vi "Advance past replacable whitespace.vi"(7 "JSON":string, 9 "Offset":i32) -> (1 "Offset of first non-whitespace":i32)   [LabVIEW 2019, in "JSONtext.lvlib"]
doc: "Advance past only whitespace that can be used in a replacement\n-- no comments, as partial replacement will cause corupt JSON"
uses:
  JSONtext.lvlib
  Parsing State.ctl
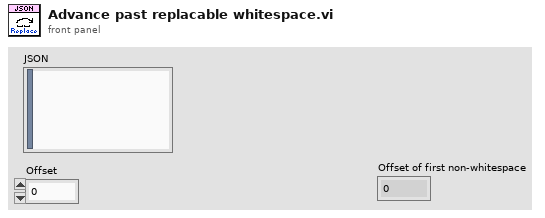
[diagram p1: front panel]
types:
  T1 = typedef "JSONtext.lvlib/Parsing State.ctl" = enum16{"Parser Error", "Object", "Array", "String", "Number/Other", "Leading Whitespace", "Object end", "Array end", "Value end"}
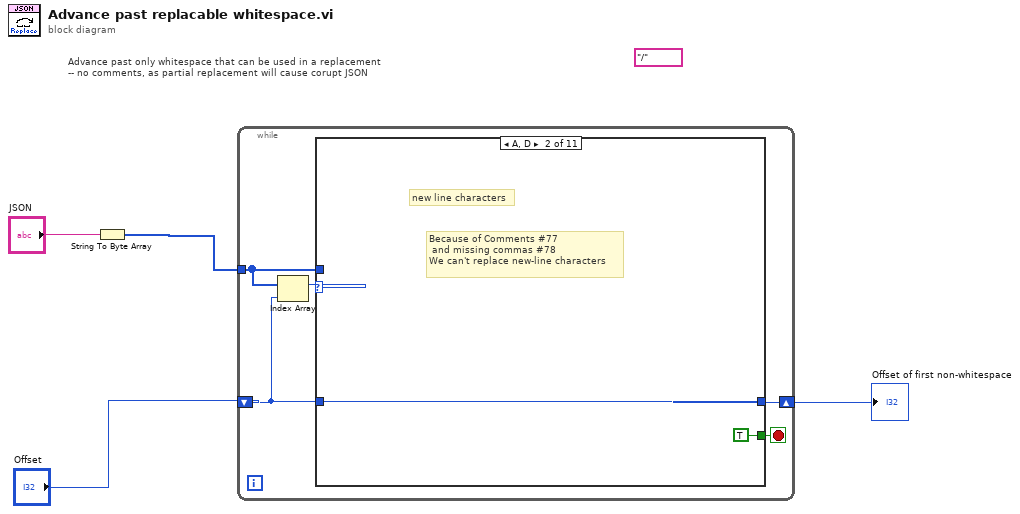
[diagram p0: block diagram]
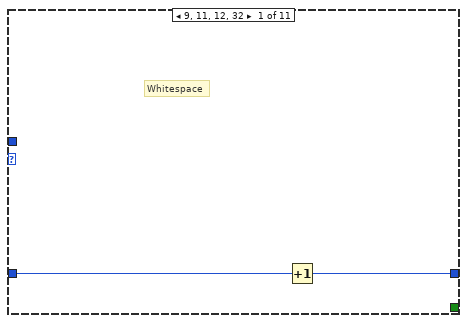
[diagram p2: hidden frame]
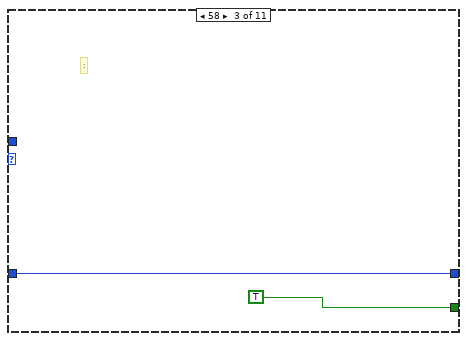
[diagram p3: hidden frame]
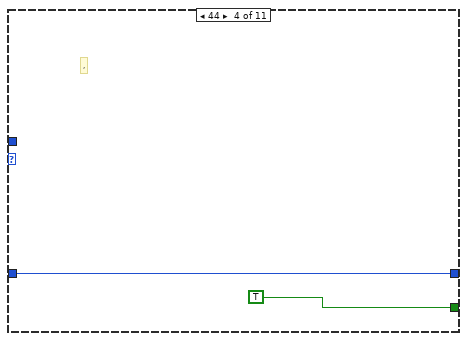
[diagram p4: hidden frame]
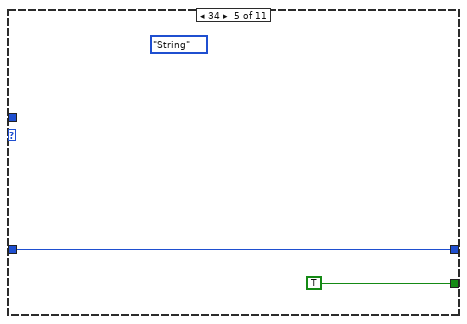
[diagram p5: hidden frame]
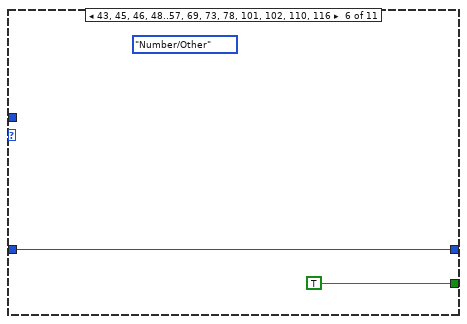
[diagram p6: hidden frame]
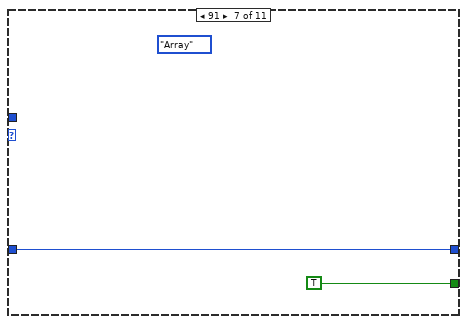
[diagram p7: hidden frame]
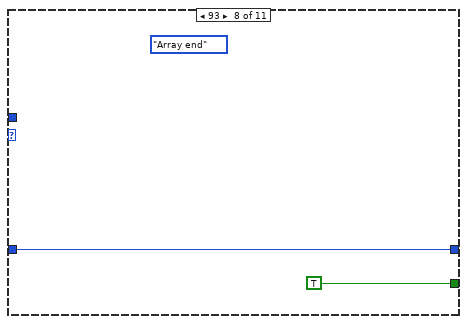
[diagram p8: hidden frame]
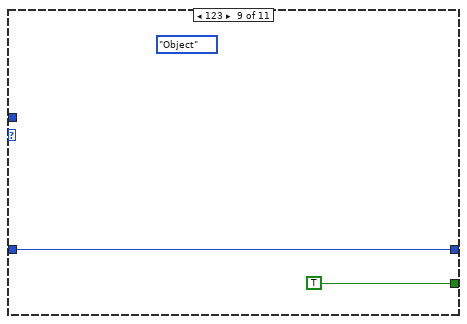
[diagram p9: hidden frame]
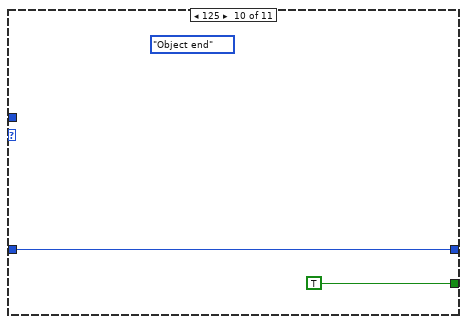
[diagram p10: hidden frame]
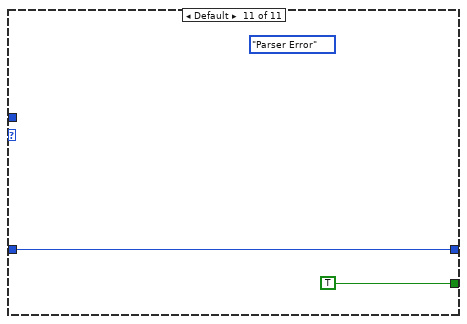
[diagram p11: hidden frame]
diagram:
  (unwired) "/"
  # "Advance past only whitespace that can be used in a replacement\n-- no comments, as partial replacement will cause corupt JSON"
  n1 = String To Byte Array(string="JSON") -> (unsigned byte array=w2:u8[])
  n2 = while {
    tunnel: w2 -> [w5]
    shift-right: [w6] -> w4
    shift-left: "Offset" -> [w7]
    stop <- w8 stop-if-true
    n3 = Index Array(array=w5, index=w7) -> (element=w9:u8)
    n4 = case shown="A, D" w9 {
      tunnel: [_ TRUE TRUE TRUE TRUE TRUE TRUE TRUE TRUE TRUE TRUE] -> w8
      tunnel: w7 -> [w11 w13 w15 w17 w18 w20 w22 w24 w26 w28 w31]
      tunnel: [w10 w13 w15 w17 w18 w20 w22 w24 w26 w28 w31] -> w6
      tunnel: w5 -> [_ _ _ _ _ _ _ _ _ _ _]
      frame 9, 11, 12, 32 {
        # "Whitespace"
        n5 = Increment(x=w11) -> (x+1=w10:i32)
      }
      frame 10, 13 {
        # "Because of Comments #77\n and missing commas #78\nWe can't replace new-line characters"
        # "new line characters"
      }
      frame 58 {
        # ":"
      }
      frame 44 {
        # ","
      }
      frame 34 {
        (unwired) Parsing_State."String"
      }
      frame 43, 45, 46, 48..57, 69, 73, 78, 101, 102, 110, 116 {
        (unwired) Parsing_State."Number/Other"
      }
      frame 91 {
        (unwired) Parsing_State."Array"
      }
      frame 93 {
        (unwired) Parsing_State."Array end"
      }
      frame 123 {
        (unwired) Parsing_State."Object"
      }
      frame 125 {
        (unwired) Parsing_State."Object end"
      }
      frame Default {
        (unwired) Parsing_State."Parser Error"
      }
    }
  }
  "Offset of first non-whitespace" <- w4
